vi "Reset Devices.vi"(0 "session in":refnum<k21>, 5 "devices":refnum<k21>="$DefaultDevices", 11 "error in (no error)":errorcluster) -> (4 "session out":refnum<k21>, 15 "error out":errorcluster)   [LabVIEW 2020, in "SLSC.lvlib"]
doc: "Resets devices to their default state. This VI sends the specified devices a hardware reset signal, reinitializes module registers to their initial value, and rereads the module's non-volatile memory. If you specify a chassis, this VI resets all of the modules in the chassis. To reboot the chassis, use the Restart VI provided by the NI System Configuration API."
uses:
  <vilib>/SLSC/SLSC.lvlib
  nislsclvapi.dll
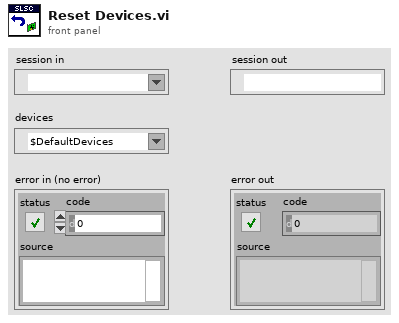
[diagram p1: front panel]
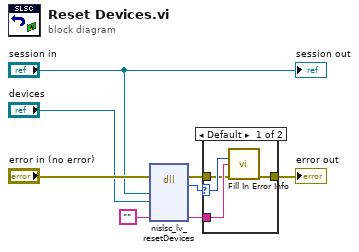
[diagram p0: block diagram]
diagram:
  n1 = dll-call lib="nislsclvapi.*" fn="nislsc_lv_resetDevices"(error in="error in (no error)", "session"="session in", "devices"="devices", "extendedErrorInfo"="") -> (error out=w4:errorcluster, "return type"=w3:i32, "extendedErrorInfo"=w5:string)  [unwired: 6 in, 1 out]
  n2 = case shown="Default" w3 {
    selector: w3 -> [w12 _]
    tunnel: w5 -> [w11 _]
    tunnel: w4 -> [w10 w13]
    tunnel: [w9 w13] -> w2
    frame Default {
      n3 = call <vilib>:"Fill In Error Info.vi"("status code"=w12, "extended error info"=w11, "error in"=w10) -> ("error out"=w9:errorcluster)  [unwired: 12 in]
    }
    frame 0 {
    }
  }
  "error out" <- w2
  "session out" <- "session in"
